vi "Prepare Results.vi"(8 "error in (no error)":errorcluster, 11 "LUnit Test Case V2 in":refnum<class "LUnit Test Case V2.lvclass">) -> (0 "error out":errorcluster, 2 "Results":T1[](array[typedef]), 3 "LUnit Test Case V2 out":refnum<class "LUnit Test Case V2.lvclass">)   [LabVIEW 2020, in "LUnit Test Case V2.lvclass"]
uses:
  LUnit Test Case V2.lvclass
  Result/Result.ctl
  Result/Status.ctl
  Result/Type.ctl
  LUnit Test Case V2.lvclass/LUnit Test Case V2.ctl
  Result/Result.lvlib
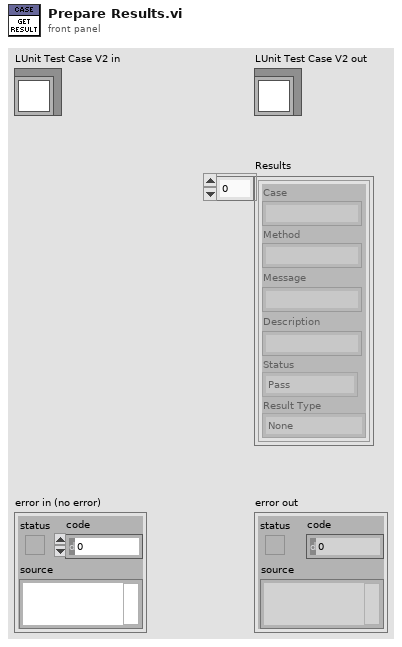
[diagram p1: front panel]
types:
  T1 = typedef "Result.lvlib/Result.ctl" = cluster{"Case":string, "Method":string, "Message":string, "Description":string, "Status":T2, "Result Type":T3}
  T2 = typedef "Result.lvlib/Status.ctl" = enum16{"Pass", "Fail", "Error", "Skipped", "Setup Error", "Broken", "Teardown Error"}
  T3 = typedef "Result.lvlib/Type.ctl" = enum16{"None", "Pass", "Fail", "Skip", "Pass if Equal", "Fail if Equal", "Pass if Error", "Fail if Error", "Pass if", "Fail if"}
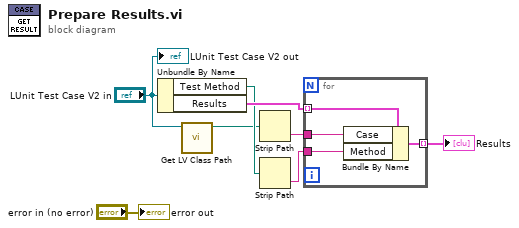
[diagram p0: block diagram]
diagram:
  n1 = Unbundle By Name("LUnit Test Case V2 in") -> ("Test Method"=w6:path, "Results"=w7:T1[])
  n2 = call <vilib>:"Get LV Class Path.vi"("object"="LUnit Test Case V2 in") -> ("class path"=w4:path)  [unwired: 9 in, 1 out]
  n3 = Strip Path(path=w4) -> (name=w3:string)  [unwired: 1 out]
  n4 = Strip Path(path=w6) -> (name=w2:string)  [unwired: 1 out]
  n5 = for {
    tunnel: w7 -> [w12] mode=indexing
    tunnel: w3 -> [w11]
    tunnel: w2 -> [w10]
    tunnel: [w9] -> w1 mode=indexing
    n6 = Bundle By Name(cluster=w12, "Case"=w11, "Method"=w10) -> (w9:T1)
  }
  "Results" <- w1
  "error out" <- "error in (no error)"
  "LUnit Test Case V2 out" <- "LUnit Test Case V2 in"
